vi "Metronome.GetBroadcasts.vi"(11 "NewTemplate in":refnum<class "Metronome.lvclass">) -> (2 "SingleLoopTemplate":cluster{"Broadcasts":T1, "Broadcasts":T2}, 3 "NewTemplate out":refnum<class "Metronome.lvclass">)   [LabVIEW 2024, in "Metronome.lvclass"]
uses:
  Metronome.lvclass
  C:/Git/JA/JQMH/RQMHCore/ModuleCore/Module.lvclass
  RQMHCore/ModuleCore/StandardBroadcasts.ctl
  RQMHCore/Shared/Died.ctl
  RQMHCore/ModuleCore/Started.ctl
  Broadcast Events--cluster.ctl
  Stopped.ctl
  RQMHCore/ModuleCore/Module.lvclass/Module.ctl
  Metronome.lvclass/Metronome.ctl
  RQMHCore/ModuleCore/Module.lvclass
  RQMHCore/Shared/ModuleShared.lvlib
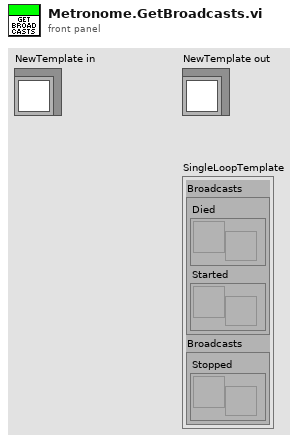
[diagram p1: front panel]
types:
  T1 = typedef "Module.lvclass/StandardBroadcasts.ctl" = cluster{"Died":refnum<user-event>, "Started":refnum<user-event>}
  T2 = typedef "Metronome.lvclass/Broadcast Events--cluster.ctl" = cluster{"Stopped":refnum<user-event>}
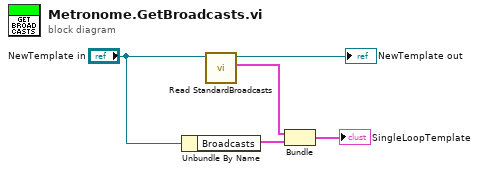
[diagram p0: block diagram]
diagram:
  n1 = Unbundle By Name("NewTemplate in") -> ("Broadcasts"=w5:T2)
  n2 = call "Read StandardBroadcasts.vi"("JQMHCore in"="NewTemplate in") -> ("Broadcasts"=w4:T1, "JQMHCore out"=→"NewTemplate out":refnum<class "Metronome.lvclass">)  [unwired: 8 in, 1 out]
  n3 = Bundle("Broadcasts"=w4, "Broadcasts"=w5) -> (→"SingleLoopTemplate":cluster{"Broadcasts":T1, "Broadcasts":T2})  [unwired: 1 in]
